vi "Main.vi"   [LabVIEW 2021]
uses:
  Ex Queue Actor/Ex Queue Actor/Ex Queue Actor.lvclass
  jettl/jettl Queue Actor/jettl Queue Actor/jettl Queue Actor.lvclass
  C:/git/jettl/src/Example/Ex Queue Actor/Ex Queue Actor/Ex Queue Actor.lvclass
  C:/git/jettl/src/Example/Pop Up/Pop Up/Pop Up.lvclass
  Actor/Queue Actor/Queue Actor.lvclass
  C:/git/jettl/src/Actor/Actor/Actor.lvclass
  C:/git/jettl/src/Actor/Msgs/Setup/Setup/Setup.lvclass
  C:/git/jettl/src/Actor/Msgs/Teardown/Teardown/Teardown.lvclass
  C:/git/jettl/src/Actor/Queue Actor/Queue Actor.lvclass
  C:/git/jettl/src/Actor/Msgs/Event Create/Event Create/Event Create.lvclass
  C:/git/jettl/src/Actor/Msgs/Event Last Ack/Event Last Ack/Event Last Ack.lvclass
  C:/git/jettl/src/Actor/Msgs/Queue Create/Queue Create/Queue Create.lvclass
  C:/git/jettl/src/Actor/Msgs/Queue Last Ack/Queue Last Ack/Queue Last Ack.lvclass
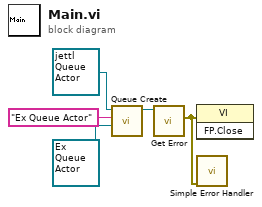
[diagram p0: block diagram]
diagram:
  n1 = call-dynamic "Queue Create.vi"("Queue Actor"=refnum<class "Ex Queue Actor.lvclass"> refnum ("Dev Actor.lvlib:Dev Actor.lvclass"), "Alias"="Ex Queue Actor", "jettl Queue Actor in"=refnum<class "jettl Queue Actor.lvclass"> refnum ("jettl Queue Actor.lvlib:jettl Queue Actor.lvclass")) -> ("jettl Queue Actor out"=w2:refnum<class "jettl Queue Actor.lvclass">)  [unwired: 8 in]
  n2 = call-dynamic "Get Error.vi"("jettl Queue Actor in"=w2) -> ("Error"=w1:errorcluster)  [unwired: 10 in]
  n3 = invoke class="VI" method="FP.Close"(error in=w1) -> ()  [unwired: 2 in, 3 out]
  n4 = call <vilib>:"Simple Error Handler.vi"("error in (no error)"=w1) -> ()  [unwired: 4 in, 5 out]
